vi "myRIO v1.2 Open Throughput AI (N Samples).vi"(7 "Allow multiple opens?":bool, 8 "error in (no error)":errorcluster, 10 "Channel Names":string[](array[string]), 11 "Resource name":T7 caption="RIO Device") -> (0 "error out":errorcluster, 1 "AI (N Samples) Scale Constants List":T1, 2 "AI (N Samples) Channel List":T3, 3 "myRIO Ref Out":T5)   [LabVIEW 2021]
uses:
  <vilib>/userDefined/High Color/nirio_resource_hc.ctl
  <vilib>/myRIO/Common/Instrument Driver Framework/Utilities/typedefs/myRIO v1.0 Reference.ctl
  <vilib>/myRIO/Common/Instrument Driver Framework/Utilities/typedefs/Generic FPGA Reference.ctl
  <vilib>/myRIO/Common/Instrument Driver Framework/myRIO v1.0/AI Block/typedefs/AI Block Channels List.ctl
  <vilib>/myRIO/Common/Instrument Driver Framework/myRIO v1.0/AI Block/typedefs/AI Block Channels Enum.ctl
  <vilib>/myRIO/Common/Instrument Driver Framework/Utilities/typedefs/Analog Scaling Constants List.ctl
  <vilib>/myRIO/Common/Instrument Driver Framework/Utilities/typedefs/Analog Scaling Constants.ctl
  <vilib>/myRIO/Common/Instrument Driver Framework/myRIO v1.0/AI Block/typedefs/myRIO v1.2 AI Block Channels Enum.ctl
  <vilib>/Utility/VariantDataType/GetNumericInfo.vi
  <vilib>/Utility/error.llb/Error Cluster From Error Code.vi
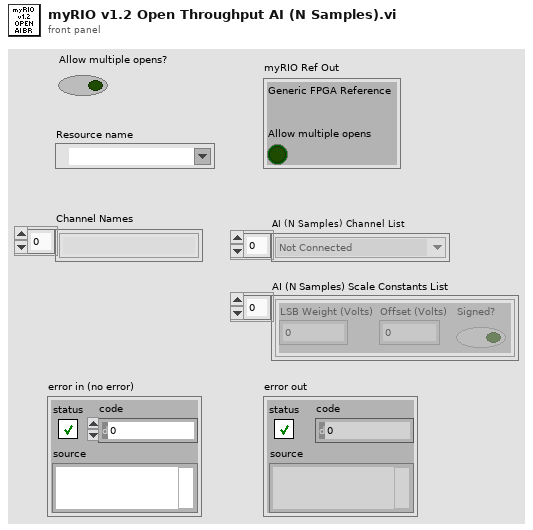
[diagram p1: front panel]
types:
  T1 = typedef "Analog Scaling Constants List.ctl" = T2[]
  T2 = typedef "Analog Scaling Constants.ctl" = cluster{"LSB Weight (Volts)":dbl, "Offset (Volts)":dbl, "Signed?":bool}
  T3 = typedef "AI Block Channels List.ctl" = T4[]
  T4 = typedef "AI Block Channels Enum.ctl" = enum16{"Not Connected", "A/AI0 (N Samples)", "A/AI1 (N Samples)", "A/AI2 (N Samples)", "A/AI3 (N Samples)", "A/AI4 (N Samples)", "A/AI5 (N Samples)", "A/AI6 (N Samples)", "A/AI7 (N Samples)", "A/AI0 (DIFF N Samples)", "A/AI1 (DIFF N Samples)", "A/AI2 (DIFF N Samples)", "A/AI3 (DIFF N Samples)", "B/AI0 (N Samples)", "B/AI1 (N Samples)", "B/AI2 (N Samples)", "B/AI3 (N Samples)", "B/AI4 (N Samples)", "B/AI5 (N Samples)", "B/AI6 (N Samples)", "B/AI7 (N Samples)", "B/AI0 (DIFF N Samples)", "B/AI1 (DIFF N Samples)", "B/AI2 (DIFF N Samples)", "B/AI3 (DIFF N Samples)"}
  T5 = typedef "myRIO v1.0 Reference.ctl" = cluster{"Generic FPGA Reference":T6, "Allow multiple opens":bool}
  T6 = typedef "Generic FPGA Reference.ctl" = refnum<k20>
  T7 = typedef "nirio_resource_hc.ctl" = tag
  T8 = typedef "myRIO v1.2 AI Block Channels Enum.ctl" = enum16{"Not Connected", "A/AI0 (N Samples)"}
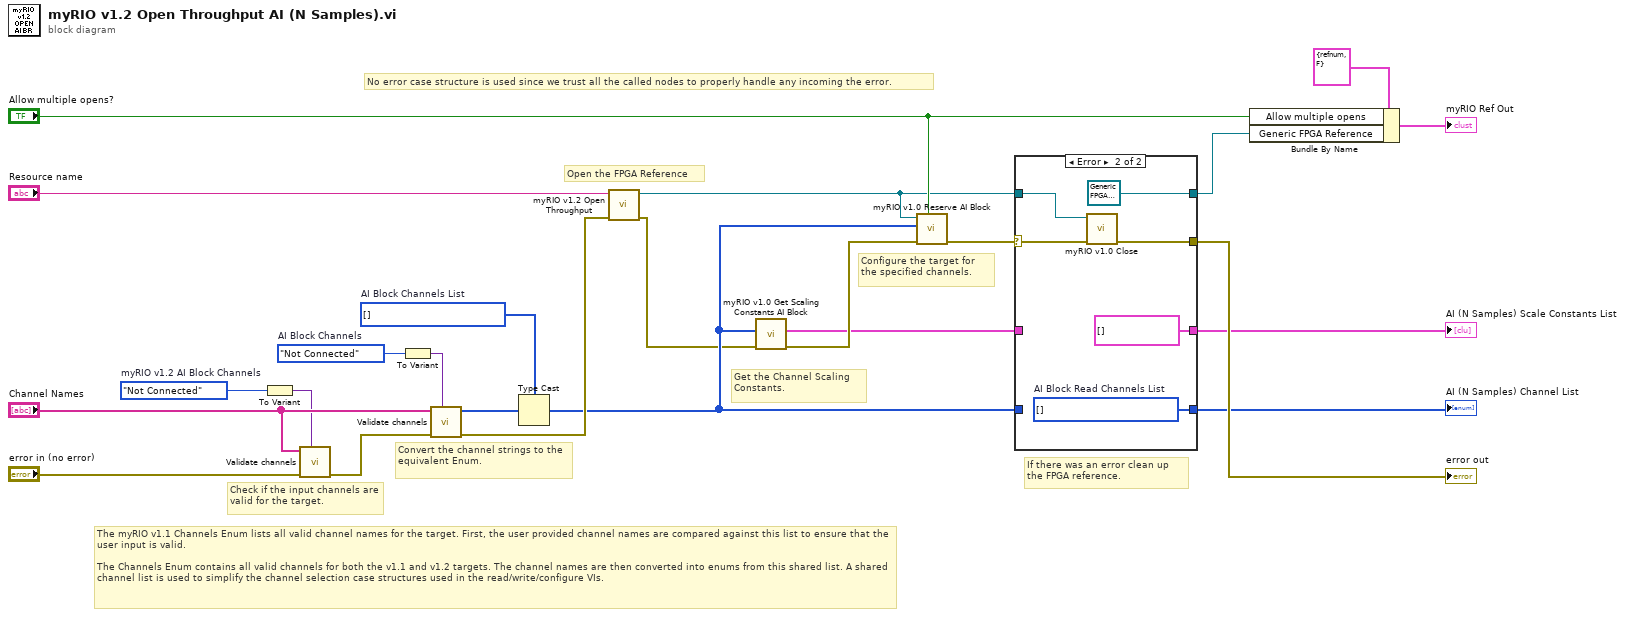
[diagram p0: block diagram]
diagram:
  w10 = T3 [] items=["Not Connected", "A/AI0 (N Samples)", "A/AI1 (N Samples)", "A/AI2 (N Samples)", "A/AI3 (N Samples)", "A/AI4 (N Samples)", "A/AI5 (N Samples)", "A/AI6 (N Samples)", "A/AI7 (N Samples)", "A/AI0 (DIFF N Samples)", "A/AI1 (DIFF N Samples)", "A/AI2 (DIFF N Samples)", "A/AI3 (DIFF N Samples)", "B/AI0 (N Samples)", "B/AI1 (N Samples)", "B/AI2 (N Samples)", "B/AI3 (N Samples)", "B/AI4 (N Samples)", "B/AI5 (N Samples)", "B/AI6 (N Samples)", "B/AI7 (N Samples)", "B/AI0 (DIFF N Samples)", "B/AI1 (DIFF N Samples)", "B/AI2 (DIFF N Samples)", "B/AI3 (DIFF N Samples)"]  # AI Block Channels List
  w11 = AI_Block_Channels_Enum."Not Connected"  # AI Block Channels
  w12 = myRIO_v1.2_AI_Block_Channels_Enum."Not Connected"  # myRIO v1.2 AI Block Channels
  # "Get the Channel Scaling Constants."
  # "The myRIO v1.1 Channels Enum lists all valid channel names for the target. First, the user provided channel names are compared against this list to ensure that the user input is valid.\n\nThe Channels Enum contains all valid channels for both the v1.1 and v1.2 targets. The channel names are then converted into enums from this shared list. A shared channel list is used to simplify the channel selection case structures used in the read/write/configure VIs."
  # "If there was an error clean up the FPGA reference."
  # "Configure the target for the specified channels."
  # "Open the FPGA Reference"
  # "No error case structure is used since we trust all the called nodes to properly handle any incoming the error."
  # "Convert the channel strings to the equivalent Enum."
  # "Check if the input channels are valid for the target."
  n1 = To Variant(anything=w12) -> (Variant=w13:variant)
  n2 = call <vilib>:"Validate channels.vi"("Channels Enum Variant"=w13, "error in (no error)"="error in (no error)", "Channel Names"="Channel Names") -> ("error out"=w23:errorcluster)  [unwired: 7 in, 1 out]
  n3 = To Variant(anything=w11) -> (Variant=w14:variant)
  n4 = call <vilib>:"Validate channels.vi"("Channels Enum Variant"=w14, "error in (no error)"=w23, "Channel Names"="Channel Names") -> ("error out"=w19:errorcluster, "Index Array"=w18:u16[])  [unwired: 7 in]
  n5 = Type Cast(type=w10, x=w18) -> (*(type *) &x=w6:T3)
  n6 = call <vilib>:"myRIO v1.2 Open Throughput.vi"("error in (no error)"=w19, "Resource name"="Resource name") -> ("error out"=w5:errorcluster, "myRIO FPGA Ref Out"=w1:T6)  [unwired: 8 in]
  n7 = call <vilib>:"myRIO v1.0 Get Scaling Constants AI Block.vi"("error in (no error)"=w5, "AI (N Samples) Channels List"=w6) -> ("error out"=w4:errorcluster, "Scale Constants Array"=w3:T1)  [unwired: 8 in]
  n8 = call <vilib>:"myRIO v1.0 Reserve AI Block.vi"("Allow multiple opens?"="Allow multiple opens?", "error in (no error)"=w4, "AI (N Samples) Channels List"=w6, "Generic FPGA Reference"=w1) -> ("error out"=w15:errorcluster)  [unwired: 7 in]
  n9 = case shown="Error" w15 {
    selector: w15 -> [w28 w34]
    tunnel: [w26 T6 refnum ("myRIO FPGA Ref Out")] -> w17
    tunnel: [w28 w33] -> w21
    tunnel: [w27 w30] -> w9
    tunnel: w6 -> [w27 _]
    tunnel: w1 -> [w26 w31]
    tunnel: w3 -> [w25 _]
    tunnel: [w25 T1 [] ("Scale Constants Array")] -> w2
    frame No Error {
    }
    frame Error {
      w30 = T3 [] items=["Not Connected", "A/AI0 (N Samples)", "A/AI1 (N Samples)", "A/AI2 (N Samples)", "A/AI3 (N Samples)", "A/AI4 (N Samples)", "A/AI5 (N Samples)", "A/AI6 (N Samples)", "A/AI7 (N Samples)", "A/AI0 (DIFF N Samples)", "A/AI1 (DIFF N Samples)", "A/AI2 (DIFF N Samples)", "A/AI3 (DIFF N Samples)", "B/AI0 (N Samples)", "B/AI1 (N Samples)", "B/AI2 (N Samples)", "B/AI3 (N Samples)", "B/AI4 (N Samples)", "B/AI5 (N Samples)", "B/AI6 (N Samples)", "B/AI7 (N Samples)", "B/AI0 (DIFF N Samples)", "B/AI1 (DIFF N Samples)", "B/AI2 (DIFF N Samples)", "B/AI3 (DIFF N Samples)"]  # AI Block Read Channels List
      n10 = call <vilib>:"myRIO v1.0 Close.vi"("error in (no error)"=w34, "myRIO FPGA Ref In"=w31) -> ("error out"=w33:errorcluster)  [unwired: 9 in]
    }
  }
  "error out" <- w21
  "AI (N Samples) Channel List" <- w9
  "AI (N Samples) Scale Constants List" <- w2
  n11 = Bundle By Name(cluster=T5 {"Generic FPGA Reference"=refnum, "Allow multiple opens"=FALSE} ("myRIO Ref Out"), "Allow multiple opens"="Allow multiple opens?", "Generic FPGA Reference"=w17) -> (→"myRIO Ref Out":T5)
